vi "ParseStartBurstModeBroadcast.vi"(8 "error in (no error)":errorcluster, 10 "msg value":variant, 11 "config":T1 {"HighPassFilterState"."Filter State" format="%.2f"; "HighPassFilterState"."IIR Filter Cluster"."Forward Coefficients" format="%.2f"; "HighPassFilterState"."IIR Filter Cluster"."Reverse Coefficients" format="%.2f"; "FixedSizeX32"."InputConfig" items=["AC Coupled", "DC Coupled", "IEPE AC Coupled"]}) -> (0 "error out":errorcluster, 3 "config out":T1 {"HighPassFilterState"."Filter State" format="%.2f"; "HighPassFilterState"."IIR Filter Cluster"."Forward Coefficients" format="%.2f"; "HighPassFilterState"."IIR Filter Cluster"."Reverse Coefficients" format="%.2f"; "FixedSizeX32"."InputConfig" items=["AC Coupled", "DC Coupled", "IEPE AC Coupled"]})   [LabVIEW 2017, in "CmsAcquisition.lvlib"]
uses:
  <vilib>/addons/InsightCM/Devices/Shared/Cms/CmsAcquisition/CmsAcquisition.lvlib
  <vilib>/addons/InsightCM/Devices/Shared/Cms/CmsAcquisition/controls/Configuration.ctl
  <vilib>/addons/InsightCM/Devices/Shared/Cms/CmsAcquisition/controls/TachometerConfig.ctl
  <vilib>/addons/InsightCM/Devices/Shared/Cms/CmsAcquisition/controls/FixedSizeArrays.ctl
  <vilib>/LabVIEW Targets/FPGA/cRIO/shared/nicrio_ModuleControls/nicrio_cRIO-9232_ConfigModeRing.ctl
  <vilib>/addons/InsightCM/Devices/Shared/Cms/cRIOWfmAcq/subVIs/RIO Wfm Cust Ctrls/rwfm_SamplingInfo.ctl
  <vilib>/addons/InsightCM/Devices/Shared/Cms/CmsAcquisition/controls/Group.ctl
  <vilib>/addons/InsightCM/Devices/Shared/Cms/CmsAcquisition/controls/Channel.ctl
  <vilib>/addons/InsightCM/Utilities/Analysis/Vibration/controls/HighPassFilterState.ctl
  <vilib>/addons/InsightCM/Devices/Shared/Cms/CmsAcquisition/controls/BurstMode.ctl
  <vilib>/addons/InsightCM/Devices/Shared/Cms/CmsBurstMode/controls/InitiateBurstMode.ctl
  <vilib>/addons/InsightCM/Devices/Shared/Cms/CmsBurstMode/BurstMode.lvlib
  <vilib>/addons/InsightCM/Devices/Shared/Cms/cRIOWfmAcq/cRIOWfmLib.lvlib
  <vilib>/addons/InsightCM/Utilities/Analysis/Vibration/VibrationAnalysisFunctions.lvlib
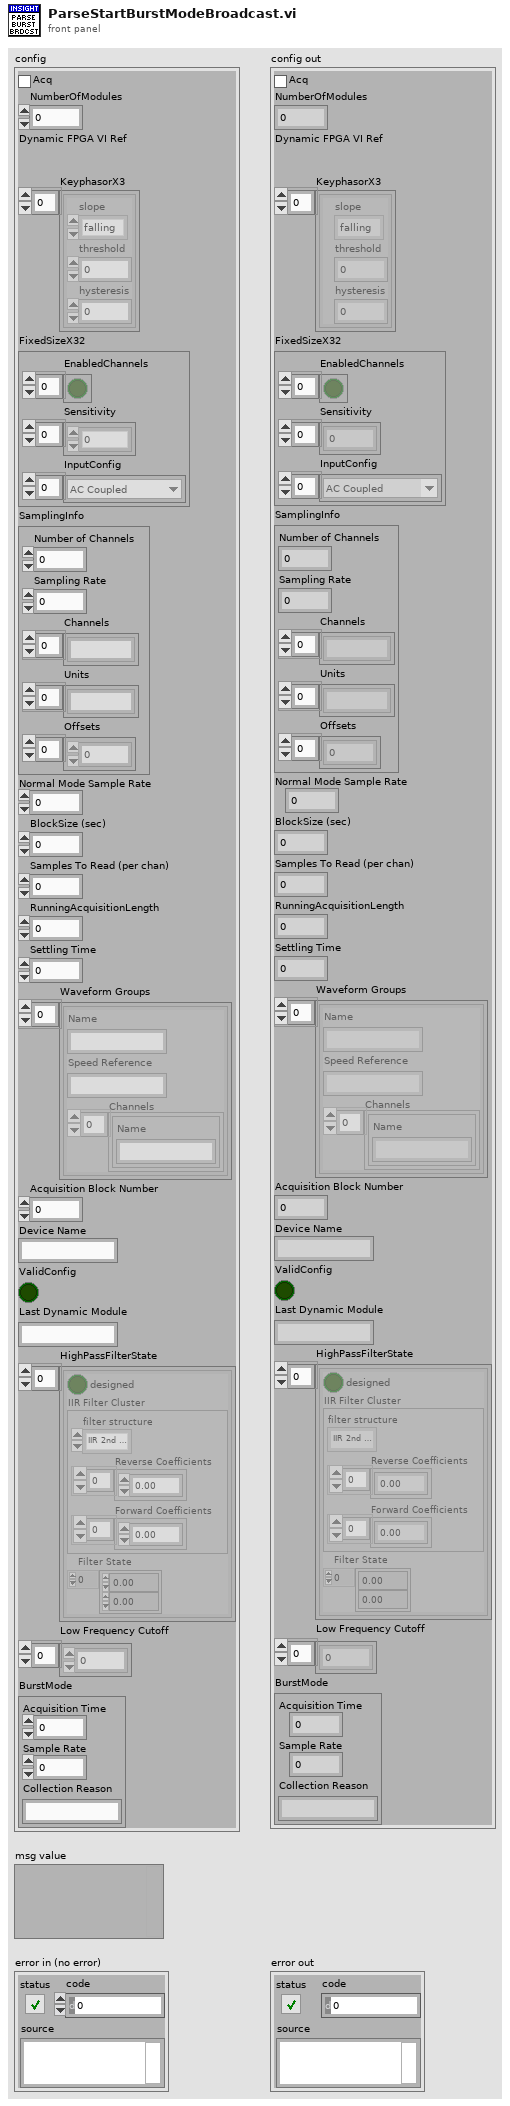
[diagram p1: front panel]
types:
  T1 = typedef "CmsAcquisition.lvlib/Configuration.ctl" = cluster{"Acq":bool, "NumberOfModules":i16, "Dynamic FPGA VI Ref":refnum<k20>, "KeyphasorX3":T2[], "FixedSizeX32":T3, "SamplingInfo":T5, "Normal Mode Sample Rate":dbl, "BlockSize (sec)":dbl, "Samples To Read (per chan)":i32, "RunningAcquisitionLength":dbl, "Settling Time":dbl, "Waveform Groups":T6[], "Acquisition Block Number":i32, "Device Name":string, "ValidConfig":bool, "Last Dynamic Module":string, "HighPassFilterState":T8[], "Low Frequency Cutoff":dbl[], "BurstMode":T9}
  T2 = typedef "CmsAcquisition.lvlib/TachometerConfig.ctl" = cluster{"slope":enum16{"falling", "rising"}, "threshold":dbl, "hysteresis":dbl}
  T3 = typedef "CmsAcquisition.lvlib/FixedSizeArrays.ctl" = cluster{"EnabledChannels":bool[], "Sensitivity":dbl[], "InputConfig":T4[]}
  T4 = typedef "nicrio_cRIO-9232_ConfigModeRing.ctl" = u8
  T5 = typedef "cRIOWfmLib.lvlib/rwfm_SamplingInfo.ctl" = cluster{"Number of Channels":i32, "Sampling Rate":dbl, "Channels":string[], "Units":string[], "Offsets":sgl[]}
  T6 = typedef "CmsAcquisition.lvlib/Group.ctl" = cluster{"Name":string, "Speed Reference":string, "Channels":T7[]}
  T7 = typedef "CmsAcquisition.lvlib/Channel.ctl" = cluster{"Name":string}
  T8 = typedef "VibrationAnalysisFunctions.lvlib/HighPassFilterState.ctl" = cluster{"designed":bool, "IIR Filter Cluster":cluster{"filter structure":enum32{"IIR 2nd Order", "IIR 4th Order"}, "Reverse Coefficients":dbl[], "Forward Coefficients":dbl[]}, "Filter State":dbl[]}
  T9 = typedef "CmsAcquisition.lvlib/BurstMode.ctl" = cluster{"Acquisition Time":dbl, "Sample Rate":dbl, "Collection Reason":string}
  T10 = typedef "BurstMode.lvlib/InitiateBurstMode.ctl" = cluster{"Group":string, "Acq Reason":string}
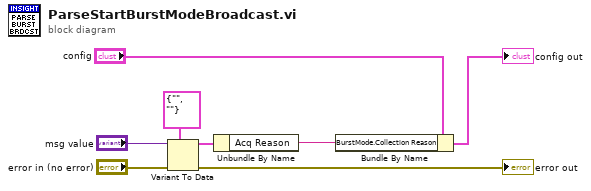
[diagram p0: block diagram]
diagram:
  n1 = Variant To Data(error in="error in (no error)", type=T10 {"Group"="", "Acq Reason"=""} ("InitiateBurstMode"), Variant="msg value") -> (data=w7:T10, error out=→"error out":errorcluster)
  n2 = Unbundle By Name(w7) -> ("Acq Reason"=w8:string)
  n3 = Bundle By Name(cluster="config", "BurstMode.Collection Reason"=w8) -> (→"config out":T1)
